vi "RestoreTreeUISettings.vi"(8 "Error In":errorcluster, 11 "UI References":T1) -> (0 "Error Out":errorcluster)   [LabVIEW 2017, in "Client.lvlib" / "UI_API.lvlib"]
uses:
  UI_API.lvlib
  TypeDefs/UIReferences.ctl
  ClientGlobals.vi
  <vilib>/Utility/config.llb/Read Key (I32).vi
  <vilib>/Utility/config.llb/Read Key (String).vi
  <vilib>/Utility/config.llb/NI_LVConfig.lvlib
  Client.lvlib
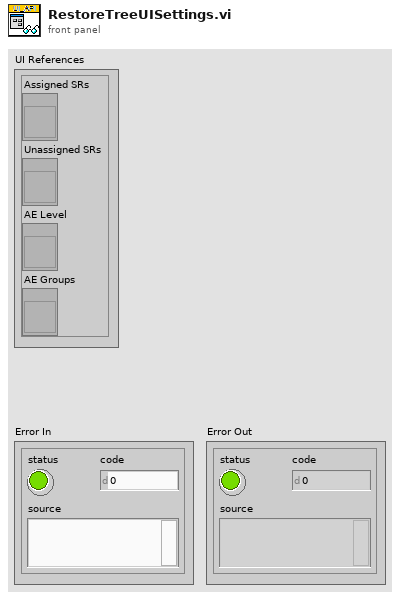
[diagram p1: front panel]
types:
  T1 = typedef "Client.lvlib/UI_API.lvlib/UIReferences.ctl" = cluster{"Assigned SRs":refnum<vi>, "Unassigned SRs":refnum<vi>, "AE Level":refnum<vi>, "AE Groups":refnum<vi>}
  T2 = typedef "NI_LVConfig.lvlib/Config Data RefNum.ctl" = refnum<k1>
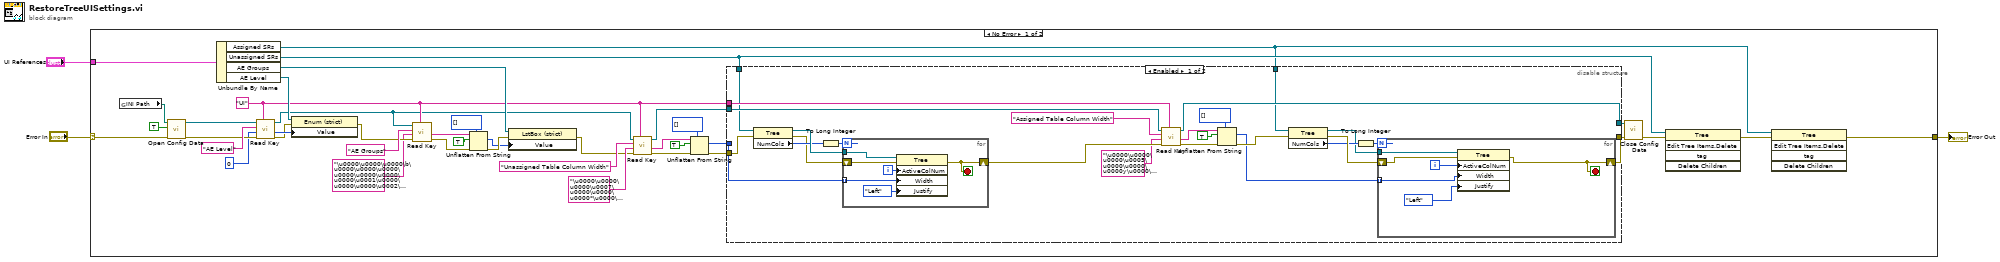
[diagram p0: block diagram]
diagram:
  n1 = case shown="No Error" "Error In" {
    selector: "Error In" -> [w42 w83]
    tunnel: "UI References" -> [w41 _]
    tunnel: [w5 w83] -> w1
    frame No Error {
      w12 = "UI" ("section")
      n2 = global read "ClientGlobals.vi" "INI Path"() -> (w4:path)
      n3 = call <vilib>:"Open Config Data.vi"("error in (no error)"=w42, "create file if necessary (T)"=TRUE ("create file if necessary? (T)"), "configuration file path"=w4) -> ("error out"=w35:errorcluster, "refnum"=w38:T2)  [unwired: 6 in, 1 out]
      n4 = Unbundle By Name(w41) -> ("Assigned SRs"=w6:refnum<vi>, "Unassigned SRs"=w8:refnum<vi>, "AE Groups"=w39:refnum<vi>, "AE Level"=w40:refnum<vi>)
      n5 = call-poly <vilib>:"Read Key.vi"("section"=w12, "error in (no error)"=w35, "default value"=0, "key"="AE Level", "refnum"=w38) -> ("error out"=w34:errorcluster, "value"=w36:i32, "refnum out"=w10:T2)  [unwired: 3 in, 1 out]
      n6 = property class="Enum (strict)"(reference=w40, error in=w34, "Value"=w36) -> (error out=w31:errorcluster)  [unwired: 1 out]
      n7 = call-poly <vilib>:"Read Key.vi"("section"=w12, "error in (no error)"=w31, "default value"="\u0000\u0000\u0000\b\u0000\u0000\u0000\u0000\u0000\u0000\u0000\u0001\u0000\u0000\u0000\u0002\u0000\u0000\u0000\u0003\u0000\u0000\u0000\u0004\u0000\u0000\u0000\u0005\u0000\u0000\u0000\u0006\u0000\u0000\u0000\u0007", "key"="AE Groups", "refnum"=w10) -> ("error out"=w28:errorcluster, "value"=w29:string)  [unwired: 3 in, 2 out]
      n8 = Unflatten From String(type=i32[] [] ("Value"), binary string=w29, data includes array or string size? (T)=TRUE, error in (no error)=w28) -> (value=w26:i32[], error out=w27:errorcluster)  [unwired: 1 in, 1 out]
      n9 = property class="LstBox (strict)"(reference=w39, error in=w27, "Value"=w26) -> (error out=w11:errorcluster)  [unwired: 1 out]
      n10 = call-poly <vilib>:"Read Key.vi"("section"=w12, "error in (no error)"=w11, "default value"="\u0000\u0000\u0000\u0007\u0000\u0000\u0000*\u0000\u0000\u0000F\u0000\u0000\u0000L\u0000\u0000\u0001\u0000\u0000\u0001\u0013\u0000\u0000\u0000E\u0000\u0000\u0000Z", "key"="Unassigned Table Column Width", "refnum"=w10) -> ("error out"=w21:errorcluster, "value"=w22:string, "refnum out"=w18:T2)  [unwired: 3 in, 1 out]
      n11 = Unflatten From String(type=u32[] [], binary string=w22, data includes array or string size? (T)=TRUE, error in (no error)=w21) -> (value=w19:u32[], error out=w20:errorcluster)  [unwired: 1 in, 1 out]
      n12 = disable-structure shown="Enabled" {
        disable-tunnel: w20 -> [w64 w81]
        disable-tunnel: w19 -> [w63 _]
        disable-tunnel: w18 -> [w60 w82]
        disable-tunnel: [w49 w81] -> w17
        disable-tunnel: [w48 w82] -> w16
        disable-tunnel: w12 -> [w46 _]
        disable-tunnel: w8 -> [w45 _]
        disable-tunnel: w6 -> [w44 _]
        frame Enabled {
          n13 = property class="Tree"(reference=w45, error in=w64) -> (reference out=w68:refnum<vi>, error out=w65:errorcluster, "NumCols"=w67:u32)
          n14 = To Long Integer(number=w67) -> (32bit integer=w66:i32)
          n15 = for {
            N: w66 -> [_]
            shift-right: [w78] -> w62
            shift-left: w65 -> [w79]
            tunnel: w68 -> [w80]
            tunnel: w63 -> [w77] mode=indexing
            i -> [w76]
            stop <- w78 stop-if-true
            n16 = property class="Tree"(reference=w80, error in=w79, "ActiveColNum"=w76, "Width"=w77, "Justify"=enum16{"Left", "Center", "Right"}."Left" ("Active Cell:Cell Justification")) -> (error out=w78:errorcluster)  [unwired: 1 out]
          }
          n17 = call-poly <vilib>:"Read Key.vi"("section"=w46, "error in (no error)"=w62, "default value"="\u0000\u0000\u0000\u0005\u0000\u0000\u0000y\u0000\u0000\u0000;\u0000\u0000\u0001n\u0000\u0000\u0001\u0000\u0000\u0001\u0013", "key"="Assigned Table Column Width", "refnum"=w60) -> ("error out"=w53:errorcluster, "value"=w52:string, "refnum out"=w48:T2)  [unwired: 3 in, 1 out]
          n18 = Unflatten From String(type=u32[] [], binary string=w52, data includes array or string size? (T)=TRUE, error in (no error)=w53) -> (value=w50:u32[], error out=w51:errorcluster)  [unwired: 1 in, 1 out]
          n19 = property class="Tree"(reference=w44, error in=w51) -> (reference out=w56:refnum<vi>, error out=w59:errorcluster, "NumCols"=w57:u32)
          n20 = To Long Integer(number=w57) -> (32bit integer=w58:i32)
          n21 = for {
            N: w58 -> [_]
            shift-right: [w72] -> w49
            shift-left: w59 -> [w73]
            tunnel: w56 -> [w74]
            tunnel: w50 -> [w70] mode=indexing
            i -> [w71]
            stop <- w72 stop-if-true
            n22 = property class="Tree"(reference=w74, error in=w73, "ActiveColNum"=w71, "Width"=w70, "Justify"=enum16{"Left", "Center", "Right"}."Left" ("Active Cell:Cell Justification")) -> (error out=w72:errorcluster)  [unwired: 1 out]
          }
        }
        frame Disabled {
        }
      }
      n23 = call <vilib>:"Close Config Data.vi"("error in (no error)"=w17, "refnum"=w16) -> ("error out"=w9:errorcluster)  [unwired: 8 in, 1 out]
      n24 = invoke on="Invoke Node" class="Tree" method="Edit Tree Items.Delete"(reference=w8, error in=w9) -> (error out=w7:errorcluster)  [unwired: 3 in, 4 out]
      n25 = invoke on="Invoke Node" class="Tree" method="Edit Tree Items.Delete"(reference=w6, error in=w7) -> (error out=w5:errorcluster)  [unwired: 3 in, 4 out]
    }
    frame Error {
    }
  }
  "Error Out" <- w1
